vi "Set Console Reply Data.vi"(8 "error in (no error)":errorcluster, 10 "Console Reply.lvclass":refnum<class "Console Reply.lvclass">, 11 "Console in":refnum<class "Console.lvclass">) -> (0 "error out":errorcluster, 3 "Console out":refnum<class "Console.lvclass">)   [LabVIEW 2015, in "EditPanel API.lvlib" / "Console.lvclass"]
uses:
  Console.lvclass
  Console Reply/Console Reply/Console Reply.lvclass
  Console.lvclass/Console.ctl
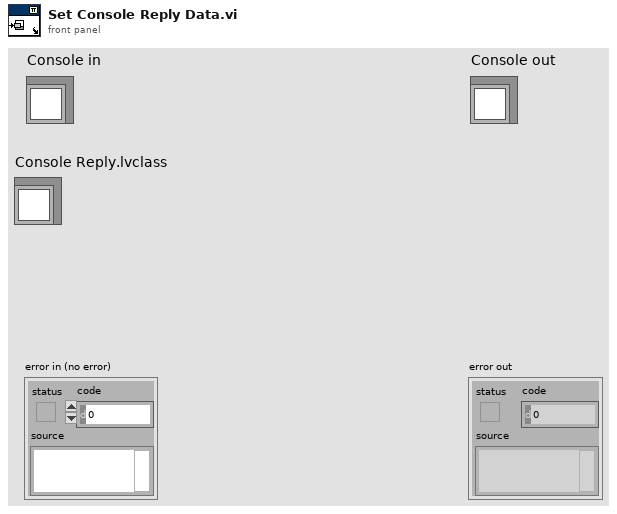
[diagram p1: front panel]
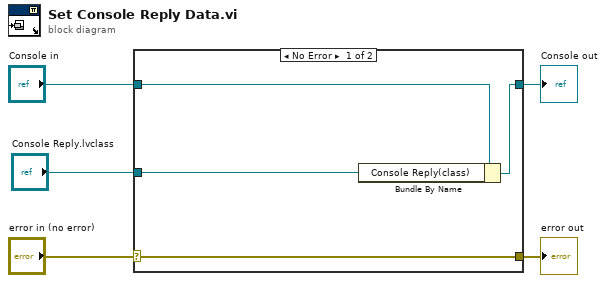
[diagram p0: block diagram]
diagram:
  n1 = case shown="No Error" "error in (no error)" {
    selector: "error in (no error)" -> [w9 w10]
    tunnel: [w9 w10] -> w4
    tunnel: [w7 w11] -> w2
    tunnel: "Console in" -> [w8 w11]
    tunnel: "Console Reply.lvclass" -> [w6 _]
    frame No Error {
      n2 = Bundle By Name(cluster=w8, "Console Reply(class)"=w6) -> (w7:refnum<class "Console.lvclass">)
    }
    frame Error {
    }
  }
  "error out" <- w4
  "Console out" <- w2
